vi "Serial only.vi"() -> ()   [LabVIEW 2016]
uses:
  <vilib>/Instr/_visa.llb/VISA Configure Serial Port (Instr).vi
panel:
  out "read buffer":string
  out "Waveform Chart":dbl(graph)
  out "Iteration":i32
  in  "Timer (ms)":u32=500
  in  "stop bits (10: 1 bit)":u16(ring)=10 items=["1.0"=10, "1.5"=15, "2.0"=20]
  in  "parity (0:none)":enum16{"None", "Odd", "Even", "Mark", "Space"}(ring)=enum."Even"
  in  "data bits (8)":u16=8
  in  "baud rate (9600)":u32=9600
  in  "VISA resource name":refnum<visa-resource-name>="COM4"
  out "field value":dbl
  in  "stop":bool
  out "error out":errorcluster
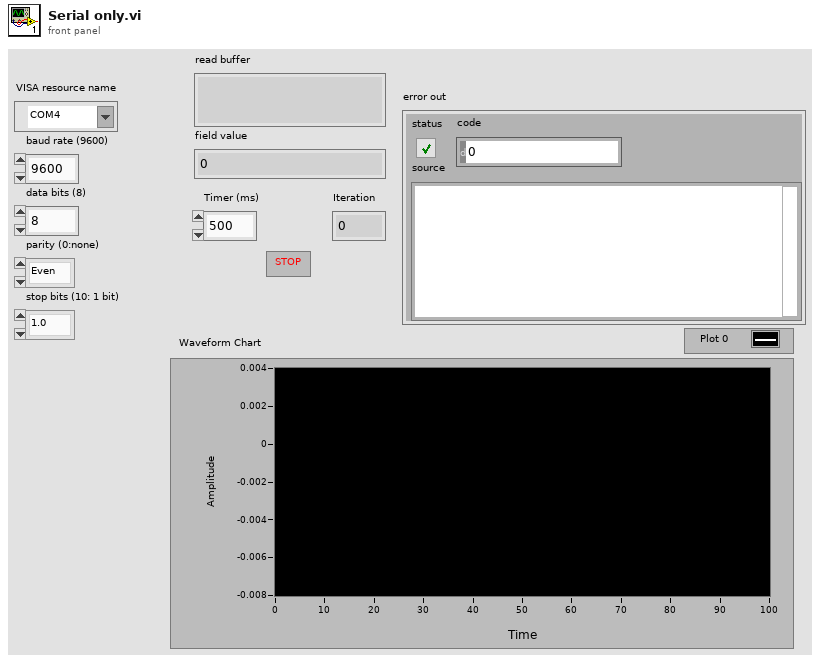
[diagram p1: front panel]
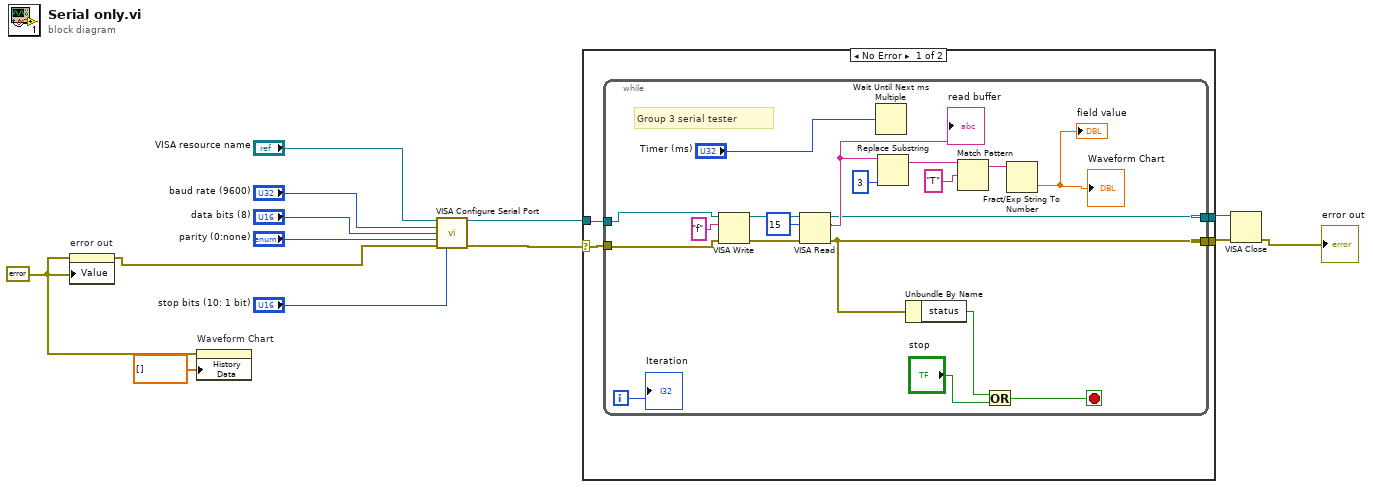
[diagram p0: block diagram]
diagram:
  w3 = errorcluster {"status"=FALSE, "code"=0, "source"=""} ("error in (no error)")
  n1 = property on="error out" class="Clust (strict)"(error in=w3, "Value"=w3) -> (error out=w4:errorcluster)  [unwired: 1 in, 1 out]
  n2 = property on="Waveform Chart" class="WFChart (strict)"(error in=w3, "History Data"=dbl[] []) -> ()  [unwired: 1 in, 2 out]
  n3 = call-poly "VISA Configure Serial Port"("VISA resource name"="VISA resource name", "baud rate (9600)"="baud rate (9600)", "data bits (8)"="data bits (8)", "parity (0:none)"="parity (0:none)", "error in (no error)"=w4, "stop bits (10: 1 bit)"="stop bits (10: 1 bit)") -> ("VISA resource name out"=w13:refnum<visa-resource-name>, "error out"=w1:errorcluster)  [unwired: 8 in]
  n4 = case shown="No Error" w1 {
    selector: w1 -> [w14 _]
    tunnel: w13 -> [w17 w38]
    tunnel: [w16 w38] -> w12
    tunnel: [w15 w37] -> w11
    frame No Error {
      n5 = while {
        tunnel: w17 -> [w32]
        tunnel: [w18] -> w16
        tunnel: w14 -> [w30]
        tunnel: [w19] -> w15
        i -> [w21]
        stop <- w34 stop-if-true
        # "Group 3 serial tester"
        n6 = VISA Write(VISA resource name=w32, write buffer="f" ("data in"), error in (no error)=w30) -> (VISA resource name out=w29:refnum<visa-resource-name>, error out=w28:errorcluster)  [unwired: 1 out]
        n7 = VISA Read(VISA resource name=w29, byte count=u32 15, error in (no error)=w28) -> (VISA resource name out=w18:refnum<visa-resource-name>, read buffer=w26:string, error out=w19:errorcluster)  [unwired: 1 out]
        "read buffer" <- w26
        n8 = Wait Until Next ms Multiple(millisecond multiple="Timer (ms)") -> ()  [unwired: 1 out]
        n9 = Replace Substring(2:3 ("length (len. of substring)"), 5:w26) -> (1:w23:string)  [unwired: 2 in, 1 out]
        n10 = Unbundle By Name(w19) -> ("status"=w35:bool)
        n11 = Match Pattern(string=w23, regular expression="T") -> (before substring=w24:string)  [unwired: 1 in, 3 out]
        n12 = Or(x=w35, y="stop") -> (x .or. y?=w34:bool)
        n13 = Fract/Exp String To Number(string=w24) -> (number=→"field value" →"Waveform Chart":dbl)  [unwired: 3 in, 1 out]
        "Iteration" <- w21
      }
    }
    frame Error {
    }
  }
  n14 = VISA Close(VISA resource name=w12, error in (no error)=w11) -> (error out=→"error out":errorcluster)
